vi "write frame to acquisition file - subvi.vi"(1 "Pixel depth":u32(ring) items=["8 bits", "16 bits", "Float", "Complex", "RGB", "HSL"], 4 "Frames per acquisition file":u32, 7 "Offset table in":cluster{"offset":i32, "file number":u8}[](array[cluster]), 8 "Error In":errorcluster, 9 "Image In":T1, 10 "Sequence files handle":T2, 11 "Last frame number written in":u32) -> (0 "Error Out":errorcluster, 2 "Last frame number written out":u32, 3 "Stop":bool, 5 "Offset table out":cluster{"offset":i32, "file number":u8}[](array[cluster]))   [LabVIEW 2014]
uses:
  <vilib>/vision/Image Controls.llb/IMAQ Image.ctl
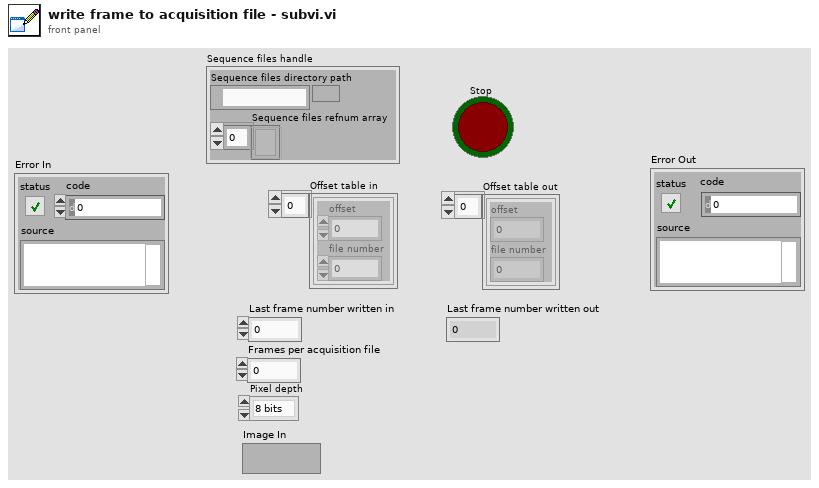
[diagram p1: front panel]
types:
  T1 = typedef "IMAQ Image.ctl" = refnum<image>
  T2 = cluster{"Sequence files directory path":path, "Sequence files refnum array":refnum<file>[]}
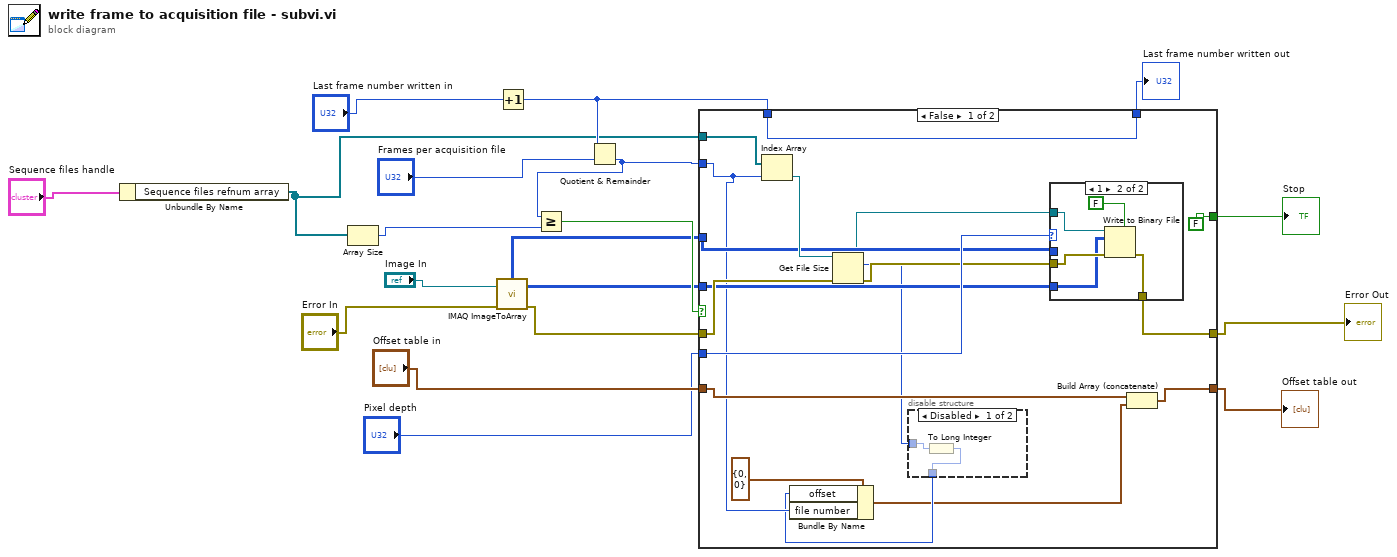
[diagram p0: block diagram]
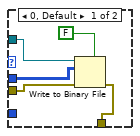
[diagram p3: hidden frame]
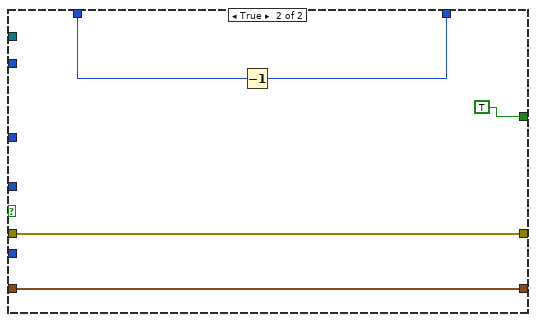
[diagram p4: hidden frame]
diagram:
  n1 = Unbundle By Name("Sequence files handle") -> ("Sequence files refnum array"=w1:refnum<file>[])
  n2 = Array Size(array=w1) -> (size(s)=w18:i32)
  n3 = call "IMAQ ImageToArray"("error in (no error)"="Error In", "Image"="Image In") -> ("error out"=w6:errorcluster, "Image Pixels (U8)"=w7:u8[][], "Image Pixels (I16)"=w8:i16[][])  [unwired: 2 in, 2 out]
  n4 = Increment(x="Last frame number written in") -> (x+1=w11:u32)
  n5 = Quotient & Remainder(x=w11, y="Frames per acquisition file") -> (floor(x/y)=w12:u32)  [unwired: 1 out]
  n6 = Greater Or Equal?(x=w12, y=w18) -> (x >= y?=w15:bool)
  n7 = case shown="False" w15 {
    tunnel: "Offset table in" -> [w28 w55]
    tunnel: "Pixel depth" -> [w33 _]
    tunnel: w12 -> [w25 _]
    tunnel: w11 -> [w36 w53]
    tunnel: w8 -> [w30 _]
    tunnel: w7 -> [w31 _]
    tunnel: w6 -> [w35 w54]
    tunnel: [w22 w55] -> w5
    tunnel: [w21 w54] -> w3
    tunnel: [w36 w52] -> w4
    tunnel: [FALSE TRUE] -> w2
    tunnel: w1 -> [w37 _]
    frame False {
      n8 = Index Array(array=w37, index=w25) -> (element=w34:refnum<file>)
      n9 = Get File Size(file=w34, error in=w35) -> (refnum out=w29:refnum<file>, size (in bytes)=w27:i64, 0:w32:errorcluster)
      n10 = disable-structure shown="Disabled" {
        disable-tunnel: w27 -> [w39 w40]
        disable-tunnel: [w38 w40] -> w24
        frame Disabled {
          n11 = To Long Integer(number=w39) -> (32bit integer=w38:i32)
        }
        frame Enabled {
        }
      }
      n12 = Bundle By Name(cluster=cluster{"offset":i32, "file number":u8} {"offset"=0, "file number"=0} ("Cluster"), "offset"=w24, "file number"=w25) -> (w23:cluster{"offset":i32, "file number":u8})
      n13 = case shown="1" w33 {
        tunnel: w32 -> [w44 w49]
        tunnel: w31 -> [w42 _]
        tunnel: w30 -> [_ w47]
        tunnel: w29 -> [w45 w50]
        tunnel: [w43 w48] -> w21
        frame 0, Default {
          n14 = Write to Binary File(file (use dialog)=w45, data=w42, error in=w44, 5:FALSE ("prepend array or string size? (T)")) -> (error out=w43:errorcluster)  [unwired: 1 in, 3 out]
        }
        frame 1 {
          n15 = Write to Binary File(file (use dialog)=w50, data=w47, error in=w49, 5:FALSE ("prepend array or string size? (T)")) -> (error out=w48:errorcluster)  [unwired: 4 out]
        }
      }
      n16 = Build Array (concatenate)(w28, w23) -> (w22:cluster{"offset":i32, "file number":u8}[])
    }
    frame True {
      n17 = Decrement(x=w53) -> (x-1=w52:u32)
    }
  }
  "Offset table out" <- w5
  "Last frame number written out" <- w4
  "Error Out" <- w3
  "Stop" <- w2
